vi "Untitled 3 (SubVI).vi"(11 "State":string) -> (1 "Color Box 3":u32(colorbox)=16448250, 2 "Color Box 2":u32(colorbox)=16448250, 3 "Color Box 1":u32(colorbox)=16448250, 4 "Color Box 4":u32(colorbox)=16448250)   [LabVIEW 2016]
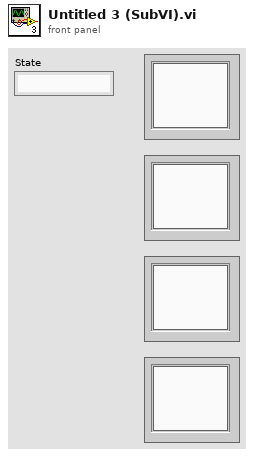
[diagram p1: front panel]
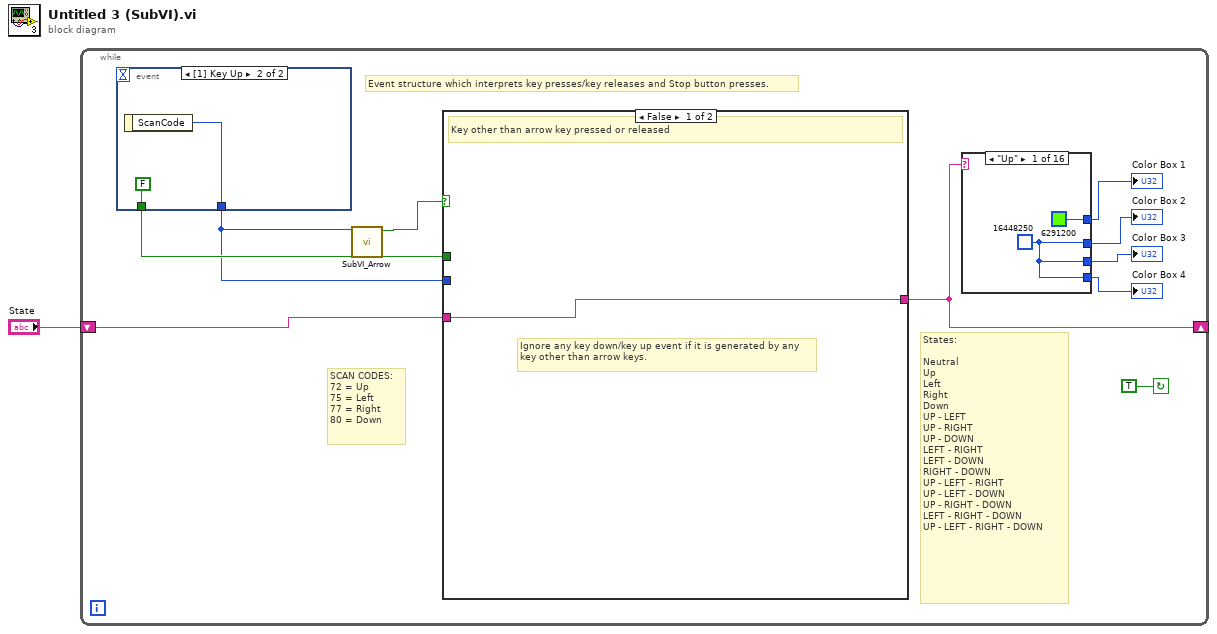
[diagram p0: block diagram]
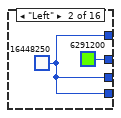
[diagram p2: hidden frame]
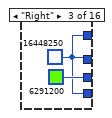
[diagram p3: hidden frame]
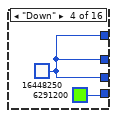
[diagram p4: hidden frame]
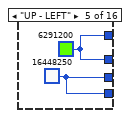
[diagram p5: hidden frame]
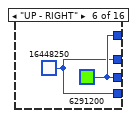
[diagram p6: hidden frame]
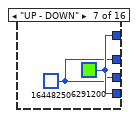
[diagram p7: hidden frame]
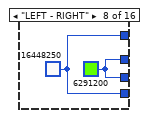
[diagram p8: hidden frame]
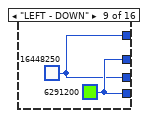
[diagram p9: hidden frame]
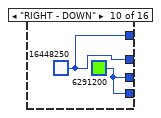
[diagram p10: hidden frame]
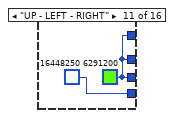
[diagram p11: hidden frame]
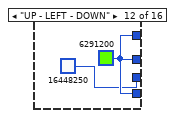
[diagram p12: hidden frame]
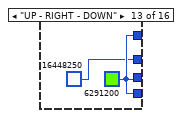
[diagram p13: hidden frame]
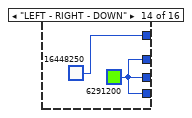
[diagram p14: hidden frame]
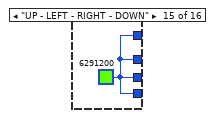
[diagram p15: hidden frame]
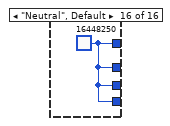
[diagram p16: hidden frame]
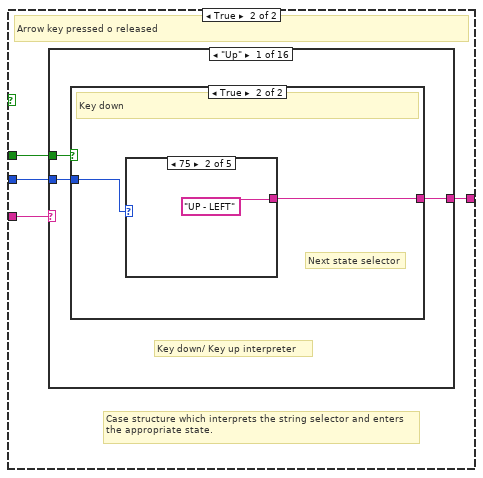
[diagram p17: hidden frame]
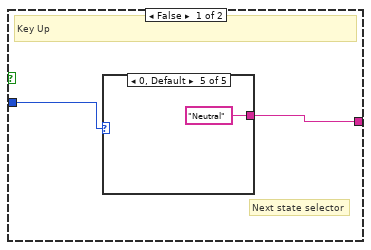
[diagram p18: hidden frame]
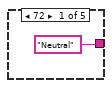
[diagram p19: hidden frame]
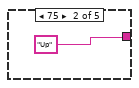
[diagram p20: hidden frame]
diagram:
  n1 = while {
    shift-right: [w9] -> _
    shift-left: "State" -> [w11]
    stop <- TRUE continue-if-true
    # "Event structure which interprets key presses/key releases and Stop button presses."
    # "States:\n\nNeutral\nUp\nLeft\nRight\nDown\nUP - LEFT\nUP - RIGHT\nUP - DOWN\nLEFT - RIGHT\nLEFT - DOWN\nRIGHT - DOWN\nUP - LEFT - RIGHT\nUP - LEFT - DOWN\nUP - RIGHT - DOWN\nLEFT - RIGHT - DOWN\nUP - LEFT - RIGHT - DOWN"
    # "SCAN CODES:\n72 = Up\n75 = Left\n77 = Right\n80 = Down"
    n2 = event shown="[1] Key Up" {
      selector: _ -> [_ _]
      dyn-events: _ -> [_ _]
      timeout: _ -> [_ _]
      tunnel: [w314 w315] -> w4
      tunnel: [TRUE FALSE] -> w10
      event Key Down {
        n3 = event-data() -> ("ScanCode"=w314:i16)  [unwired: 1 in]
      }
      event Key Up {
        n4 = event-data() -> ("ScanCode"=w315:i16)  [unwired: 1 in]
      }
    }
    n5 = call "SubVI_Arrow.vi"("ScanCode"=w4) -> ("Arrow key"=w3:bool)  [unwired: 10 in]
    n6 = case shown="False" w3 {
      tunnel: w11 -> [w42 w46]
      tunnel: w10 -> [_ w45]
      tunnel: w4 -> [_ w44]
      tunnel: [w42 w43] -> w9
      frame False {
        # "Ignore any key down/key up event if it is generated by any key other than arrow keys."
        # "Key other than arrow key pressed or released"
      }
      frame True {
        # "Case structure which interprets the string selector and enters the appropriate state."
        # "Arrow key pressed o released"
        n7 = case shown="\"Up\"" w46 {
          tunnel: w45 -> [w49 w66 w83 w100 w117 w134 w151 w168 w185 w202 w219 w236 w253 w270 w287 w304]
          tunnel: w44 -> [w48 w65 w82 w99 w116 w133 w150 w167 w184 w201 w218 w235 w252 w269 w286 w303]
          tunnel: [w47 w64 w81 w98 w115 w132 w149 w166 w183 w200 w217 w234 w251 w268 w285 w302] -> w43
          frame "Up" {
            # "Key down/ Key up interpreter"
            n8 = case shown="True" w49 {
              tunnel: w48 -> [w51 w58]
              tunnel: [w50 w57] -> w47
              frame False {
                # "Next state selector"
                # "Key Up"
                n9 = case shown="0, Default" w51 {
                  tunnel: ["Neutral" ("State") "Up" ("State") "Up" ("State") "Up" ("State") "Neutral" ("State")] -> w50
                  frame 72 {
                  }
                  frame 75 {
                  }
                  frame 77 {
                  }
                  frame 80 {
                  }
                  frame 0, Default {
                  }
                }
              }
              frame True {
                # "Next state selector"
                # "Key down"
                n10 = case shown="75" w58 {
                  tunnel: ["Up" ("State") "UP - LEFT" ("State") "UP - RIGHT" ("State") "UP - DOWN" ("State") "Neutral" ("State")] -> w57
                  frame 72 {
                  }
                  frame 75 {
                  }
                  frame 77 {
                  }
                  frame 80 {
                  }
                  frame 0, Default {
                  }
                }
              }
            }
          }
          frame "Left" {
            n11 = case shown="True" w66 {
              tunnel: w65 -> [w68 w75]
              tunnel: [w67 w74] -> w64
              frame False {
                # "Key Up"
                n12 = case shown="80" w68 {
                  tunnel: ["Left" ("State") "Neutral" ("State") "Left" ("State") "Left" ("State") "Neutral" ("State")] -> w67
                  frame 72 {
                  }
                  frame 75 {
                  }
                  frame 77 {
                  }
                  frame 80 {
                  }
                  frame 0, Default {
                  }
                }
              }
              frame True {
                # "Key down"
                n13 = case shown="0, Default" w75 {
                  tunnel: ["UP - LEFT" ("State") "Left" ("State") "LEFT - RIGHT" ("State") "LEFT - DOWN" ("State") "Neutral" ("State")] -> w74
                  frame 72 {
                  }
                  frame 75 {
                  }
                  frame 77 {
                  }
                  frame 80 {
                  }
                  frame 0, Default {
                  }
                }
              }
            }
          }
          frame "Right" {
            n14 = case shown="True" w83 {
              tunnel: w82 -> [w85 w92]
              tunnel: [w84 w91] -> w81
              frame False {
                # "Key Up"
                n15 = case shown="80" w85 {
                  tunnel: ["Right" ("State") "Right" ("State") "Neutral" ("State") "Right" ("State") "Neutral" ("State")] -> w84
                  frame 72 {
                  }
                  frame 75 {
                  }
                  frame 77 {
                  }
                  frame 80 {
                  }
                  frame 0, Default {
                  }
                }
              }
              frame True {
                # "Key down"
                n16 = case shown="0, Default" w92 {
                  tunnel: ["UP - RIGHT" ("State") "LEFT - RIGHT" ("State") "Right" ("State") "RIGHT - DOWN" ("State") "Neutral" ("State")] -> w91
                  frame 72 {
                  }
                  frame 75 {
                  }
                  frame 77 {
                  }
                  frame 80 {
                  }
                  frame 0, Default {
                  }
                }
              }
            }
          }
          frame "Down" {
            n17 = case shown="True" w100 {
              tunnel: w99 -> [w102 w109]
              tunnel: [w101 w108] -> w98
              frame False {
                # "Key Up"
                n18 = case shown="80" w102 {
                  tunnel: ["Down" ("State") "Down" ("State") "Down" ("State") "Neutral" ("State") "Neutral" ("State")] -> w101
                  frame 72 {
                  }
                  frame 75 {
                  }
                  frame 77 {
                  }
                  frame 80 {
                  }
                  frame 0, Default {
                  }
                }
              }
              frame True {
                # "Key down"
                n19 = case shown="72" w109 {
                  tunnel: ["UP - DOWN" ("State") "LEFT - DOWN" ("State") "RIGHT - DOWN" ("State") "Down" ("State") "Neutral" ("State")] -> w108
                  frame 72 {
                  }
                  frame 75 {
                  }
                  frame 77 {
                  }
                  frame 80 {
                  }
                  frame 0, Default {
                  }
                }
              }
            }
          }
          frame "UP - LEFT" {
            n20 = case shown="False" w117 {
              tunnel: w116 -> [w119 w126]
              tunnel: [w118 w125] -> w115
              frame False {
                # "Key Up"
                n21 = case shown="80" w119 {
                  tunnel: ["Left" ("State") "Up" ("State") "UP - LEFT" ("State") "UP - LEFT" ("State") "Neutral" ("State")] -> w118
                  frame 72 {
                  }
                  frame 75 {
                  }
                  frame 77 {
                  }
                  frame 80 {
                  }
                  frame 0, Default {
                  }
                }
              }
              frame True {
                # "Key down"
                n22 = case shown="0, Default" w126 {
                  tunnel: ["UP - LEFT" ("State") "UP - LEFT" ("State") "UP - LEFT - RIGHT" ("State") "UP - LEFT - DOWN" ("State") "Neutral" ("State")] -> w125
                  frame 72 {
                  }
                  frame 75 {
                  }
                  frame 77 {
                  }
                  frame 80 {
                  }
                  frame 0, Default {
                  }
                }
              }
            }
          }
          frame "UP - RIGHT" {
            n23 = case shown="True" w134 {
              tunnel: w133 -> [w136 w143]
              tunnel: [w135 w142] -> w132
              frame False {
                # "Key Up"
                n24 = case shown="0, Default" w136 {
                  tunnel: ["Right" ("State") "UP - RIGHT" ("State") "Up" ("State") "UP - RIGHT" ("State") "Neutral" ("State")] -> w135
                  frame 72 {
                  }
                  frame 75 {
                  }
                  frame 77 {
                  }
                  frame 80 {
                  }
                  frame 0, Default {
                  }
                }
              }
              frame True {
                # "Key down"
                n25 = case shown="0, Default" w143 {
                  tunnel: ["UP - RIGHT" ("State") "UP - LEFT - RIGHT" ("State") "UP - RIGHT" ("State") "UP - RIGHT - DOWN" ("State") "Neutral" ("State")] -> w142
                  frame 72 {
                  }
                  frame 75 {
                  }
                  frame 77 {
                  }
                  frame 80 {
                  }
                  frame 0, Default {
                  }
                }
              }
            }
          }
          frame "UP - DOWN" {
            n26 = case shown="True" w151 {
              tunnel: w150 -> [w153 w160]
              tunnel: [w152 w159] -> w149
              frame False {
                # "Key Up"
                n27 = case shown="0, Default" w153 {
                  tunnel: ["Down" ("State") "UP - DOWN" ("State") "UP - DOWN" ("State") "Up" ("State") "Neutral" ("State")] -> w152
                  frame 72 {
                  }
                  frame 75 {
                  }
                  frame 77 {
                  }
                  frame 80 {
                  }
                  frame 0, Default {
                  }
                }
              }
              frame True {
                # "Key down"
                n28 = case shown="75" w160 {
                  tunnel: ["UP - DOWN" ("State") "UP - LEFT - DOWN" ("State") "UP - RIGHT - DOWN" ("State") "UP - DOWN" ("State") "Neutral" ("State")] -> w159
                  frame 72 {
                  }
                  frame 75 {
                  }
                  frame 77 {
                  }
                  frame 80 {
                  }
                  frame 0, Default {
                  }
                }
              }
            }
          }
          frame "LEFT - RIGHT" {
            n29 = case shown="False" w168 {
              tunnel: w167 -> [w170 w177]
              tunnel: [w169 w176] -> w166
              frame False {
                # "Key Up"
                n30 = case shown="80" w170 {
                  tunnel: ["LEFT - RIGHT" ("State") "Right" ("State") "Left" ("State") "LEFT - RIGHT" ("State") "Neutral" ("State")] -> w169
                  frame 72 {
                  }
                  frame 75 {
                  }
                  frame 77 {
                  }
                  frame 80 {
                  }
                  frame 0, Default {
                  }
                }
              }
              frame True {
                # "Key down"
                n31 = case shown="80" w177 {
                  tunnel: ["UP - LEFT - RIGHT" ("State") "LEFT - RIGHT" ("State") "LEFT - RIGHT" ("State") "LEFT - RIGHT - DOWN" ("State") "Neutral" ("State")] -> w176
                  frame 72 {
                  }
                  frame 75 {
                  }
                  frame 77 {
                  }
                  frame 80 {
                  }
                  frame 0, Default {
                  }
                }
              }
            }
          }
          frame "LEFT - DOWN" {
            n32 = case shown="False" w185 {
              tunnel: w184 -> [w187 w194]
              tunnel: [w186 w193] -> w183
              frame False {
                # "Key Up"
                n33 = case shown="80" w187 {
                  tunnel: ["LEFT - DOWN" ("State") "Down" ("State") "LEFT - DOWN" ("State") "Left" ("State") "Neutral" ("State")] -> w186
                  frame 72 {
                  }
                  frame 75 {
                  }
                  frame 77 {
                  }
                  frame 80 {
                  }
                  frame 0, Default {
                  }
                }
              }
              frame True {
                # "Key down"
                n34 = case shown="0, Default" w194 {
                  tunnel: ["UP - LEFT - DOWN" ("State") "LEFT - DOWN" ("State") "LEFT - RIGHT - DOWN" ("State") "LEFT - DOWN" ("State") "Neutral" ("State")] -> w193
                  frame 72 {
                  }
                  frame 75 {
                  }
                  frame 77 {
                  }
                  frame 80 {
                  }
                  frame 0, Default {
                  }
                }
              }
            }
          }
          frame "RIGHT - DOWN" {
            n35 = case shown="True" w202 {
              tunnel: w201 -> [w204 w211]
              tunnel: [w203 w210] -> w200
              frame False {
                # "Key Up"
                n36 = case shown="0, Default" w204 {
                  tunnel: ["RIGHT - DOWN" ("State") "RIGHT - DOWN" ("State") "Down" ("State") "Right" ("State") "Neutral" ("State")] -> w203
                  frame 72 {
                  }
                  frame 75 {
                  }
                  frame 77 {
                  }
                  frame 80 {
                  }
                  frame 0, Default {
                  }
                }
              }
              frame True {
                # "Key down"
                n37 = case shown="0, Default" w211 {
                  tunnel: ["UP - RIGHT - DOWN" ("State") "LEFT - RIGHT - DOWN" ("State") "RIGHT - DOWN" ("State") "RIGHT - DOWN" ("State") "Neutral" ("State")] -> w210
                  frame 72 {
                  }
                  frame 75 {
                  }
                  frame 77 {
                  }
                  frame 80 {
                  }
                  frame 0, Default {
                  }
                }
              }
            }
          }
          frame "UP - LEFT - RIGHT" {
            n38 = case shown="True" w219 {
              tunnel: w218 -> [w221 w228]
              tunnel: [w220 w227] -> w217
              frame False {
                # "Key Up"
                n39 = case shown="0, Default" w221 {
                  tunnel: ["LEFT - RIGHT" ("State") "UP - RIGHT" ("State") "UP - LEFT" ("State") "UP - LEFT - RIGHT" ("State") "Neutral" ("State")] -> w220
                  frame 72 {
                  }
                  frame 75 {
                  }
                  frame 77 {
                  }
                  frame 80 {
                  }
                  frame 0, Default {
                  }
                }
              }
              frame True {
                # "Key down"
                n40 = case shown="0, Default" w228 {
                  tunnel: ["UP - LEFT - RIGHT" ("State") "UP - LEFT - RIGHT" ("State") "UP - LEFT - RIGHT" ("State") "UP - LEFT - RIGHT - DOWN" ("State") "Neutral" ("State")] -> w227
                  frame 72 {
                  }
                  frame 75 {
                  }
                  frame 77 {
                  }
                  frame 80 {
                  }
                  frame 0, Default {
                  }
                }
              }
            }
          }
          frame "UP - LEFT - DOWN" {
            n41 = case shown="True" w236 {
              tunnel: w235 -> [w238 w245]
              tunnel: [w237 w244] -> w234
              frame False {
                # "Key Up"
                n42 = case shown="80" w238 {
                  tunnel: ["LEFT - DOWN" ("State") "UP - DOWN" ("State") "UP - LEFT - DOWN" ("State") "UP - LEFT" ("State") "Neutral" ("State")] -> w237
                  frame 72 {
                  }
                  frame 75 {
                  }
                  frame 77 {
                  }
                  frame 80 {
                  }
                  frame 0, Default {
                  }
                }
              }
              frame True {
                # "Key down"
                n43 = case shown="80" w245 {
                  tunnel: ["UP - LEFT - DOWN" ("State") "UP - LEFT - DOWN" ("State") "UP - LEFT - RIGHT - DOWN" ("State") "UP - LEFT - DOWN" ("State") "Neutral" ("State")] -> w244
                  frame 72 {
                  }
                  frame 75 {
                  }
                  frame 77 {
                  }
                  frame 80 {
                  }
                  frame 0, Default {
                  }
                }
              }
            }
          }
          frame "UP - RIGHT - DOWN" {
            n44 = case shown="True" w253 {
              tunnel: w252 -> [w255 w262]
              tunnel: [w254 w261] -> w251
              frame False {
                # "Key Up"
                n45 = case shown="0, Default" w255 {
                  tunnel: ["RIGHT - DOWN" ("State") "UP - RIGHT - DOWN" ("State") "UP - DOWN" ("State") "UP - RIGHT" ("State") "Neutral" ("State")] -> w254
                  frame 72 {
                  }
                  frame 75 {
                  }
                  frame 77 {
                  }
                  frame 80 {
                  }
                  frame 0, Default {
                  }
                }
              }
              frame True {
                # "Key down"
                n46 = case shown="0, Default" w262 {
                  tunnel: ["UP - RIGHT - DOWN" ("State") "UP - LEFT - RIGHT - DOWN" ("State") "UP - RIGHT - DOWN" ("State") "UP - RIGHT - DOWN" ("State") "Neutral" ("State")] -> w261
                  frame 72 {
                  }
                  frame 75 {
                  }
                  frame 77 {
                  }
                  frame 80 {
                  }
                  frame 0, Default {
                  }
                }
              }
            }
          }
          frame "LEFT - RIGHT - DOWN" {
            n47 = case shown="False" w270 {
              tunnel: w269 -> [w272 w279]
              tunnel: [w271 w278] -> w268
              frame False {
                # "Key Up"
                n48 = case shown="80" w272 {
                  tunnel: ["LEFT - RIGHT - DOWN" ("State") "RIGHT - DOWN" ("State") "LEFT - DOWN" ("State") "LEFT - RIGHT" ("State") "Neutral" ("State")] -> w271
                  frame 72 {
                  }
                  frame 75 {
                  }
                  frame 77 {
                  }
                  frame 80 {
                  }
                  frame 0, Default {
                  }
                }
              }
              frame True {
                # "Key down"
                n49 = case shown="80" w279 {
                  tunnel: ["UP - LEFT - RIGHT - DOWN" ("State") "LEFT - RIGHT - DOWN" ("State") "LEFT - RIGHT - DOWN" ("State") "LEFT - RIGHT - DOWN" ("State") "Neutral" ("State")] -> w278
                  frame 72 {
                  }
                  frame 75 {
                  }
                  frame 77 {
                  }
                  frame 80 {
                  }
                  frame 0, Default {
                  }
                }
              }
            }
          }
          frame "UP - LEFT - RIGHT - DOWN" {
            n50 = case shown="False" w287 {
              tunnel: w286 -> [w289 w296]
              tunnel: [w288 w295] -> w285
              frame False {
                # "Key Up"
                n51 = case shown="80" w289 {
                  tunnel: ["LEFT - RIGHT - DOWN" ("State") "UP - RIGHT - DOWN" ("State") "UP - LEFT - DOWN" ("State") "UP - LEFT - RIGHT" ("State") "Neutral" ("State")] -> w288
                  frame 72 {
                  }
                  frame 75 {
                  }
                  frame 77 {
                  }
                  frame 80 {
                  }
                  frame 0, Default {
                  }
                }
              }
              frame True {
                # "Key down"
                n52 = case shown="80" w296 {
                  tunnel: ["UP - LEFT - RIGHT - DOWN" ("State") "UP - LEFT - RIGHT - DOWN" ("State") "UP - LEFT - RIGHT - DOWN" ("State") "UP - LEFT - RIGHT - DOWN" ("State") "Neutral" ("State")] -> w295
                  frame 72 {
                  }
                  frame 75 {
                  }
                  frame 77 {
                  }
                  frame 80 {
                  }
                  frame 0, Default {
                  }
                }
              }
            }
          }
          frame "Neutral", Default {
            n53 = case shown="True" w304 {
              tunnel: w303 -> [_ w307]
              tunnel: ["Neutral" ("State") w306] -> w302
              frame False {
                # "Key Up"
              }
              frame True {
                # "Next state selector"
                # "Key down"
                n54 = case shown="0, Default" w307 {
                  tunnel: ["Neutral" ("State") "Up" ("State") "Left" ("State") "Right" ("State") "Down" ("State")] -> w306
                  frame 0, Default {
                  }
                  frame 72 {
                  }
                  frame 75 {
                  }
                  frame 77 {
                  }
                  frame 80 {
                  }
                }
              }
            }
          }
        }
      }
    }
    n55 = case shown="\"Up\"" w9 {
      tunnel: [u32 6291200 ("Color Box 2") w14 w16 w18 w21 w23 w25 w26 w28 w30 w33 w35 w37 u32 16448250 ("Color Box 2") w40 w41] -> w8
      tunnel: [w12 u32 6291200 ("Color Box 2") w16 w18 w21 w22 w24 w27 w29 w30 w33 w35 u32 16448250 ("Color Box 2") w39 w40 w41] -> w7
      tunnel: [w12 w14 u32 6291200 ("Color Box 2") w18 w20 w23 w24 w27 w28 w31 w33 u32 16448250 ("Color Box 2") w37 w39 w40 w41] -> w6
      tunnel: [w12 w14 w16 u32 6291200 ("Color Box 2") w20 w22 w25 w26 w29 w31 u32 16448250 ("Color Box 2") w35 w37 w39 w40 w41] -> w5
      frame "Up" {
        w12 = u32 16448250 ("Color Box 2")
      }
      frame "Left" {
        w14 = u32 16448250 ("Color Box 2")
      }
      frame "Right" {
        w16 = u32 16448250 ("Color Box 2")
      }
      frame "Down" {
        w18 = u32 16448250 ("Color Box 2")
      }
      frame "UP - LEFT" {
        w21 = u32 6291200 ("Color Box 2")
        w20 = u32 16448250 ("Color Box 2")
      }
      frame "UP - RIGHT" {
        w23 = u32 6291200 ("Color Box 2")
        w22 = u32 16448250 ("Color Box 2")
      }
      frame "UP - DOWN" {
        w25 = u32 6291200 ("Color Box 2")
        w24 = u32 16448250 ("Color Box 2")
      }
      frame "LEFT - RIGHT" {
        w27 = u32 6291200 ("Color Box 2")
        w26 = u32 16448250 ("Color Box 2")
      }
      frame "LEFT - DOWN" {
        w29 = u32 6291200 ("Color Box 2")
        w28 = u32 16448250 ("Color Box 2")
      }
      frame "RIGHT - DOWN" {
        w31 = u32 6291200 ("Color Box 2")
        w30 = u32 16448250 ("Color Box 2")
      }
      frame "UP - LEFT - RIGHT" {
        w33 = u32 6291200 ("Color Box 2")
      }
      frame "UP - LEFT - DOWN" {
        w35 = u32 6291200 ("Color Box 2")
      }
      frame "UP - RIGHT - DOWN" {
        w37 = u32 6291200 ("Color Box 2")
      }
      frame "LEFT - RIGHT - DOWN" {
        w39 = u32 6291200 ("Color Box 2")
      }
      frame "UP - LEFT - RIGHT - DOWN" {
        w40 = u32 6291200 ("Color Box 2")
      }
      frame "Neutral", Default {
        w41 = u32 16448250 ("Color Box 2")
      }
    }
    "Color Box 2" <- w7
    "Color Box 3" <- w6
    "Color Box 4" <- w5
    "Color Box 1" <- w8
  }
